vi "Msg.vi"(7 "jettl in":refnum<class "jettl.lvclass">, 11 "Last Ack Created Msg Strategy in":refnum<class "Last Ack Created Msg Strategy.lvclass">) -> (5 "jettl out":refnum<class "jettl.lvclass">)   [LabVIEW 2021, in "jettl.lvlib" / "Last Ack Created Msg Strategy.lvlib" / "Last Ack Created Msg Strategy.lvclass"]
uses:
  Last Ack Created Msg Strategy.lvclass
  Last Ack Created Msg Strategy.lvclass/Last Ack Created Msg Strategy.ctl
  Last Ack Created/Last Ack Created.lvclass
  jettl/jettl.lvclass
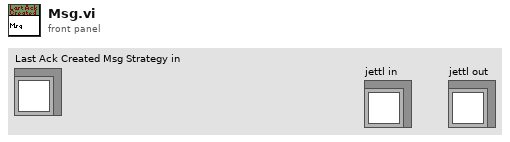
[diagram p1: front panel]
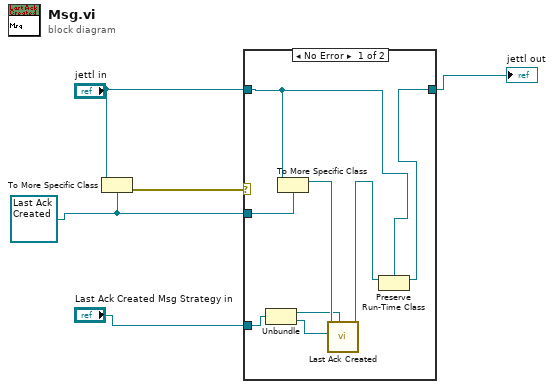
[diagram p0: block diagram]
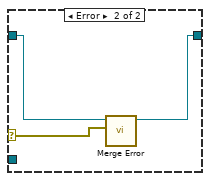
[diagram p2: hidden frame]
diagram:
  w3 = refnum<class "Last Ack Created.lvclass"> refnum ("Last Ack.lvlib:Last Ack.lvclass")
  n1 = To More Specific Class(target class=w3, reference="jettl in") -> (error out=w5:errorcluster)  [unwired: 1 in, 1 out]
  n2 = case shown="No Error" w5 {
    selector: w5 -> [_ w16]
    tunnel: [w8 w14] -> w1
    tunnel: "jettl in" -> [w10 w15]
    tunnel: w3 -> [w13 _]
    tunnel: "Last Ack Created Msg Strategy in" -> [w11 _]
    frame No Error {
      n3 = Unbundle "Unbundle"(w11) -> (w7:refnum<class "Sender.lvclass">, w6:refnum<class "jettl.lvclass">)
      n4 = To More Specific Class(target class=w13, reference=w10) -> (specific class reference=w12:refnum<class "Last Ack Created.lvclass">)  [unwired: 1 in, 1 out]
      n5 = call-dynamic "Last Ack Created.vi"("Sender"=w7, "jettl"=w6, "Last Ack Created in"=w12) -> ("Last Ack Created out"=w9:refnum<class "Last Ack Created.lvclass">)  [unwired: 8 in]
      n6 = Preserve Run-Time Class(object in=w9, 2:w10) -> (object out=w8:refnum<class "jettl.lvclass">)  [unwired: 1 in, 1 out]
    }
    frame Error {
      n7 = call-dynamic "Merge Error.vi"("Error"=w16, "Merge Error in"=w15) -> ("Merge Error out"=w14:refnum<class "jettl.lvclass">)  [unwired: 9 in]
    }
  }
  "jettl out" <- w1
